vi "Mean.vi"(7 "trial_number":i64, 8 "feature_number":i64, 11 "Target/NonTarget":dbl[][](array[numeric])) -> (3 "mean":dbl[](array[numeric]))   [LabVIEW 2014]
uses:
  <vilib>/Analysis/baseanly.llb/Mean (DBL).vi
  <vilib>/Analysis/NI_AALBase.lvlib
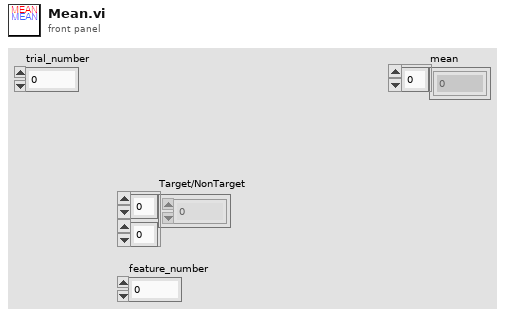
[diagram p1: front panel]
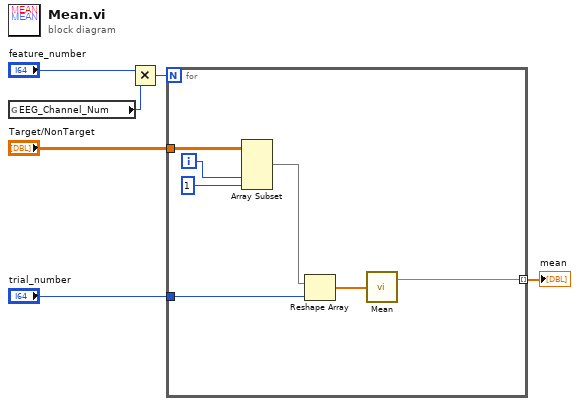
[diagram p0: block diagram]
diagram:
  n1 = global read "Control_Panel.vi" "EEG_Channel_Num"() -> (w1:i32)
  n2 = Multiply(x="feature_number", y=w1) -> (x*y=w3:i64)
  n3 = for {
    N: w3 -> [_]
    tunnel: "Target/NonTarget" -> [w13]
    tunnel: "trial_number" -> [w7]
    tunnel: [w10] -> w4 mode=indexing
    i -> [w8]
    n4 = Array Subset(array=w13, index (col)=w8, length (col)=1 ("length")) -> (w12:dbl[][])  [unwired: 2 in]
    n5 = Reshape Array(w12, w7) -> (w11:dbl[])
    n6 = call-poly <vilib>:"Mean.vi"("X"=w11) -> ("mean"=w10:dbl)  [unwired: 1 out]
  }
  "mean" <- w4
